vi "getWavelengthNoDisp.vi"(0 "Done":bool, 1 "OK Button":bool) -> ()   [LabVIEW 2016]
uses:
  <vilib>/Analysis/baseanly.llb/Mean (DBL).vi
  <vilib>/Utility/file.llb/Write Delimited Spreadsheet (DBL).vi
  <vilib>/Analysis/NI_AALBase.lvlib
  x32/CLDevIFace.dll
panel:
  out "date string":string
  in  "Folder path input":path=path "C:/Users/Lab/Desktop/Data/Wavemeter"
  out "Time":dbl
  out "Wavelength":dbl format="%0.5f"
  in  "Avg":i32=1
  out "Power (mW)":dbl format="%.9f"
  in  "Delay Time (s)":dbl=0.01
  out "error out":errorcluster
  out "output param":i32
  in  "CommPort":dbl=5.0 caption="Comm Port #"
  # "Pr = 605.977 nm"
  # "Super cavity FSR  6 GHz\nZerodure FSR  750 MHz"
  # "1 pm = 200 MHz @1212nm\n1 pm = 800 MHz @606 nm"
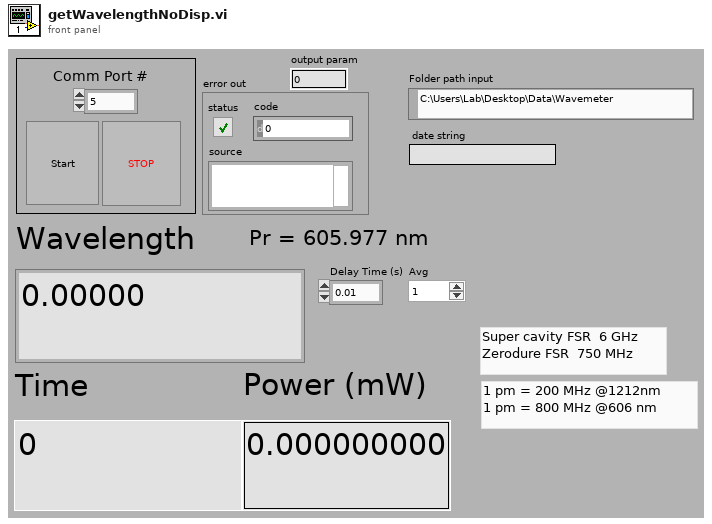
[diagram p1: front panel]
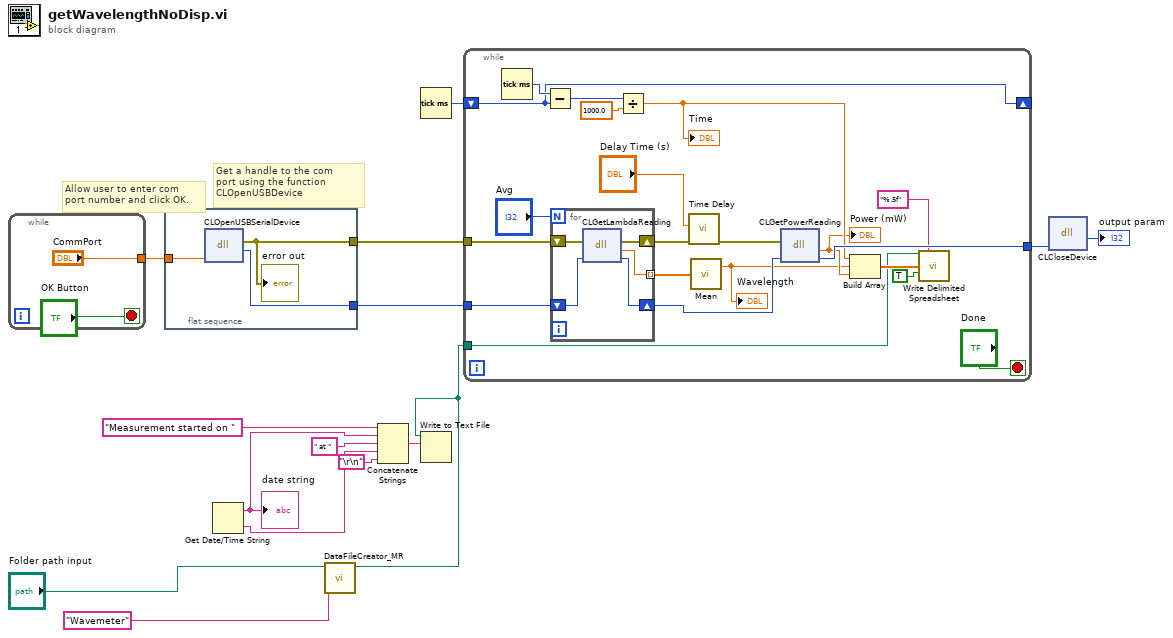
[diagram p0: block diagram]
diagram:
  # "Get a handle to the com\nport using the function CLOpenUSBDevice"
  # "Allow user to enter com \nport number and click OK."
  n1 = while {
    tunnel: ["CommPort"] -> w15
    stop <- "OK Button" stop-if-true
  }
  n2 = flat-sequence {
    tunnel: w15 -> [w20]
    tunnel: [w19] -> w14
    tunnel: [w18] -> w11
    frame #0 {
      n3 = dll-call lib="C:/Users/Lab/Desktop/AFCgit/AFC-code/HardWare/LabView/Wavemeter/x32/CLDevIFace.dll" fn="CLOpenUSBSerialDevice"("commPort"=w20) -> (error out=w18:errorcluster, "return type"=w19:i32)  [unwired: 4 in, 1 out]
      "error out" <- w18
    }
  }
  n4 = Get Date/Time String() -> (date string=w4:string, time string=w7:string)  [unwired: 3 in]
  "date string" <- w4
  n5 = call "DataFileCreator_MR.vi"("ProjectName"="Wavemeter", "Folder path input"="Folder path input") -> ("NewFilePath"=w1:path)  [unwired: 8 in, 1 out]
  n6 = Concatenate Strings("Measurement started on ", w4, " at " ("string"), w7, "\r\n") -> (w6:string)
  n7 = Tick Count (ms)() -> (millisecond timer value=w10:u32)
  n8 = Write to Text File(file (use dialog)=w1, text=w6) -> ()  [unwired: 2 in, 3 out]
  n9 = while {
    tunnel: w14 -> [w41]
    tunnel: [w35] -> w13
    tunnel: w11 -> [w38]
    shift-right: [w29] -> _
    shift-left: w10 -> [w29]
    tunnel: w1 -> [w26]
    stop <- "Done" stop-if-true
    n10 = Tick Count (ms)() -> (millisecond timer value=w32:u32)
    n11 = Subtract(x=w32, y=w29) -> (x-y=w30:u32)
    n12 = for {
      N: "Avg" -> [_]
      tunnel: [w45] -> w33 mode=indexing
      shift-right: [w42] -> w36
      shift-left: w41 -> [w46]
      shift-right: [w44] -> w39
      shift-left: w38 -> [w43]
      n13 = dll-call lib="C:/Users/Lab/Desktop/AFCgit/AFC-code/HardWare/LabView/Wavemeter/x32/CLDevIFace.dll" fn="CLGetLambdaReading"(error in=w43, "devHandle"=w46) -> (error out=w44:errorcluster, "return type"=w45:dbl, "devHandle"=w42:i32)  [unwired: 2 in, 1 out]
    }
    n14 = Divide(x=w30, y=1000.0) -> (x/y=w28:dbl)
    "Time" <- w28
    n15 = call "Time Delay"("error in (no error)"=w39, "Delay Time (s)"="Delay Time (s)") -> ("error out"=w37:errorcluster)  [unwired: 9 in]
    n16 = call-poly <vilib>:"Mean.vi"("X"=w33) -> ("mean"=w22:dbl)  [unwired: 1 out]
    "Wavelength" <- w22
    n17 = dll-call lib="C:/Users/Lab/Desktop/AFCgit/AFC-code/HardWare/LabView/Wavemeter/x32/CLDevIFace.dll" fn="CLGetPowerReading"(error in=w37, "devHandle"=w36) -> ("return type"=w23:dbl, "devHandle"=w35:i32)  [unwired: 2 in, 2 out]
    "Power (mW)" <- w23
    n18 = Build Array(w28, w22, w23) -> (w27:dbl[])
    n19 = call-poly <vilib>:"Write Delimited Spreadsheet.vi"("file path (dialog if empty)"=w26, "format (%.3f)"="%.5f", "1D data"=w27, "append to file? (new file:F)"=TRUE) -> ()  [unwired: 10 in, 2 out]
  }
  n20 = dll-call lib="C:/Users/Lab/Desktop/AFCgit/AFC-code/HardWare/LabView/Wavemeter/x32/CLDevIFace.dll" fn="CLCloseDevice"("commPort"=w13) -> ("return type"=→"output param":i32)  [unwired: 4 in, 2 out]
